vi "Wash Display Console View.vi"(8 "error in (no error)":errorcluster, 11 "View Model":T2) -> (0 "error out":errorcluster)   [LabVIEW 2017]
doc: "The interface via wich the wash controller displays the progres of the car wash.\n[Covers: UI3]"
uses:
  View Model/Controls/View Model.ctl
  View Model/Controls/Shared Model.ctl
  Error Handler/Controls/Error Model.ctl
  Error Handler/Controls/Error Data.ctl
  Error Handler/Controls/Error Level.ctl
  Configuration/Controls/Config Model.ctl
  Configuration/Controls/Config Record.ctl
  Configuration/Controls/Config Data.ctl
  Configuration/Controls/Config Command.ctl
  Controller/Controls/Controler Model.ctl
  Entry Console View/Controls/Entry Console - Wash Steps.ctl
  Controller/Controls/Controller - Overhead.ctl
  Controller/Controls/Controller - States.ctl
  Controller/Controls/Controller - Wash Step.ctl
  Vehicle Position View/Controls/Vehicle - Station Enum.ctl
  Controller/Controls/Controller - Event.ctl
  Controller/Controls/Controller - Commands.ctl
panel:
  out "Time Remaining":dbl format="%07.2g"
  out "Wash Entry":bool
  out "Vehicle Out of Position":bool
  out "Car Wash Indicators":T1
  # "Seconds"
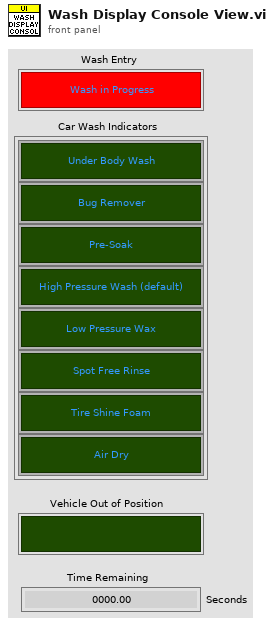
[diagram p1: front panel]
types:
  T1 = typedef "Entry Console - Wash Steps.ctl" = cluster{"Under Body Wash":bool, "Bug Remover":bool, "Pre-Soak":bool, "High Pressure Wash":bool, "Low Pressure Wax":bool, "Spot Free Rinse":bool, "Tire Shine Foam":bool, "Air Dry":bool}
  T2 = typedef "View Model.ctl" = cluster{"Shared Model":T3, "Error Model":T4, "Config Model":T5, "Controler Model":T6}
  T3 = typedef "Shared Model.ctl" = cluster{"Stop":refnum<user-event>, "Stop DVR":refnum<data-value>}
  T4 = typedef "Error Model.ctl" = cluster{"Error":refnum<user-event>}
  T5 = typedef "Config Model.ctl" = cluster{"Config Recs DVR":refnum<data-value>, "Config Data":refnum<user-event>, "Config Lock":refnum<user-event>, "Config Lock DVR":refnum<data-value>}
  T6 = typedef "Controler Model.ctl" = cluster{"Wash Step Exec":refnum<user-event>, "Wash Step Complete":refnum<user-event>, "Wash Cycle Complete":refnum<user-event>, "Wash Cycle Start":refnum<user-event>, "Vehicle Out of Position":refnum<user-event>, "Overhead DVR":refnum<data-value>, "Start Wash Step":refnum<user-event>, "Station Change":refnum<user-event>, "Command":refnum<user-event>}
  T7 = typedef "Controller - Wash Step.ctl" = enum16{"Under Body Wash", "Bug Remover", "Pre-Soak", "High Pressure Wash", "Low Pressure Wax", "Spot Free Rinse", "Tire Shine Foam", "Air Dry"}
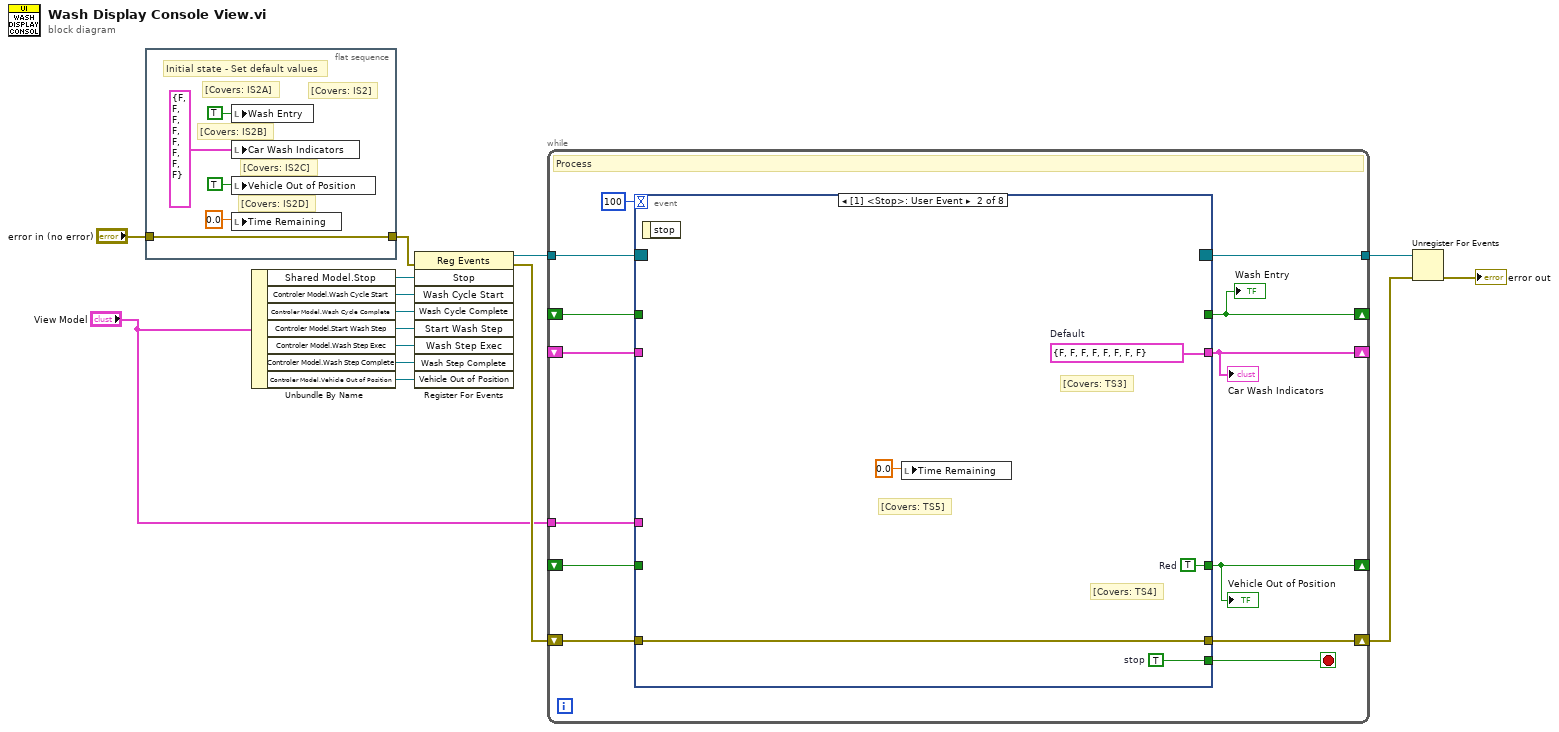
[diagram p0: block diagram]
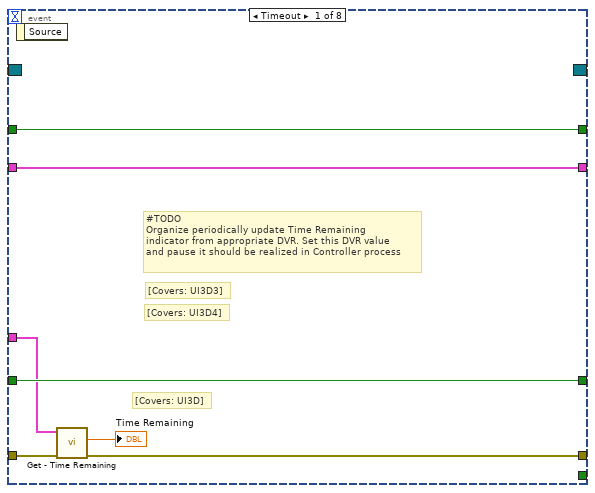
[diagram p2: hidden frame]
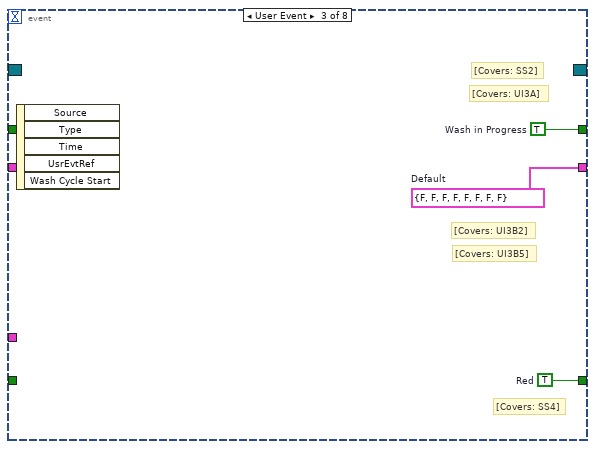
[diagram p3: hidden frame]
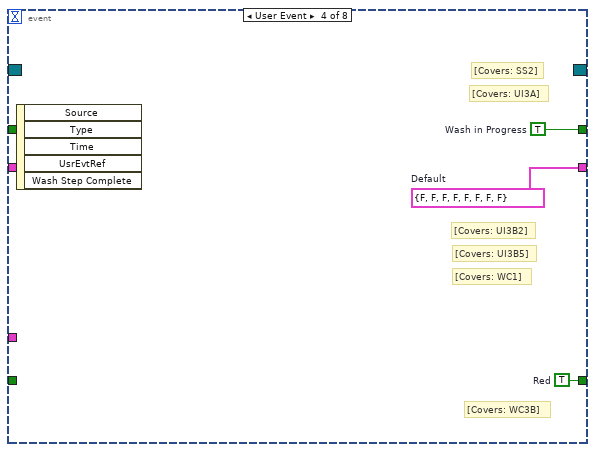
[diagram p4: hidden frame]
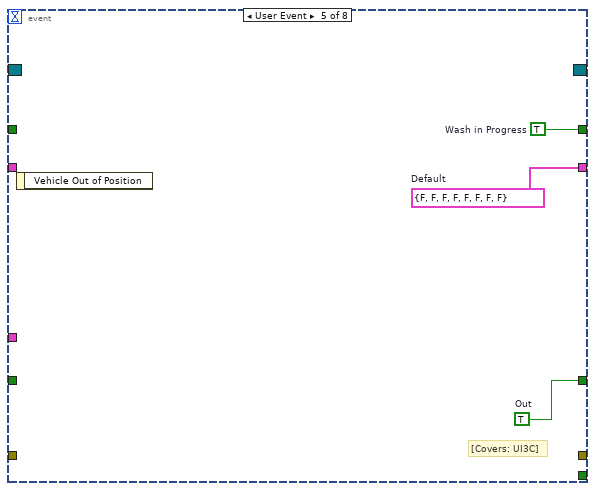
[diagram p5: hidden frame]
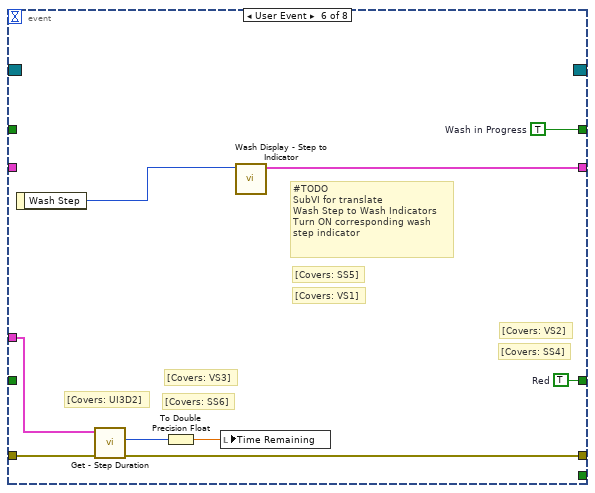
[diagram p6: hidden frame]
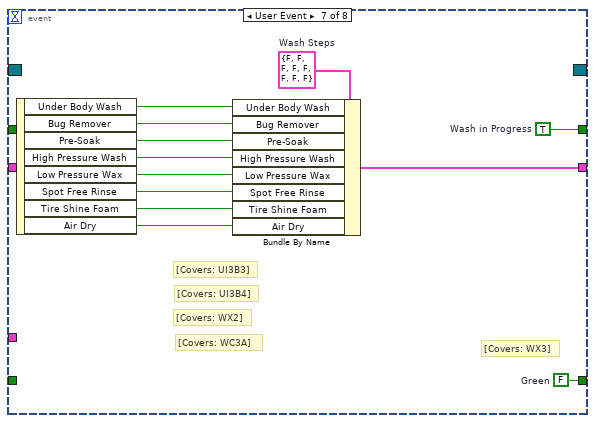
[diagram p7: hidden frame]
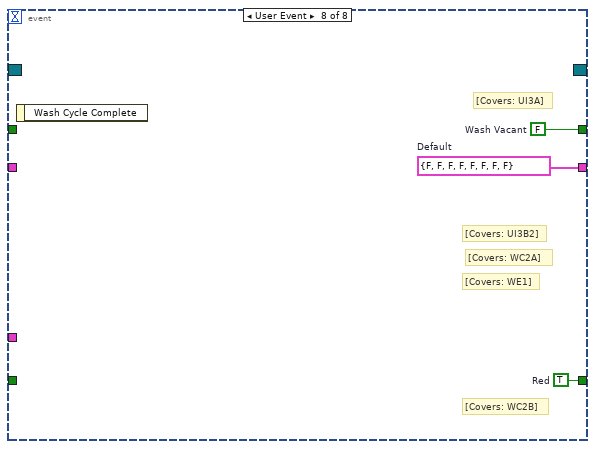
[diagram p8: hidden frame]
diagram:
  n1 = flat-sequence {
    tunnel: "error in (no error)" -> [w20]
    tunnel: [w20] -> w1
    frame #0 {
      # "[Covers: IS2D]"
      # "[Covers: IS2C]"
      # "[Covers: IS2B]"
      # "[Covers: IS2A]"
      # "[Covers: IS2]"
      # "Initial state - Set default values"
      n2 = local write "Wash Entry"(TRUE ("Wash Entry")) -> ()
      n3 = local write "Car Wash Indicators"(T1 {"Under Body Wash"=FALSE, "Bug Remover"=FALSE, "Pre-Soak"=FALSE, "High Pressure Wash"=FALSE, "Low Pressure Wax"=FALSE, "Spot Free Rinse"=FALSE, "Tire Shine Foam"=FALSE, "Air Dry"=FALSE} ("Car Wash Indicators")) -> ()
      n4 = local write "Vehicle Out of Position"(TRUE ("Vehicle Out of Position")) -> ()
      n5 = local write "Time Remaining"(0.0 ("Time Remaining")) -> ()
    }
  }
  n6 = Unbundle By Name("View Model") -> ("Shared Model.Stop"=w15:refnum<user-event>, "Controler Model.Wash Cycle Start"=w8:refnum<user-event>, "Controler Model.Wash Cycle Complete"=w7:refnum<user-event>, "Controler Model.Start Wash Step"=w4:refnum<user-event>, "Controler Model.Wash Step Exec"=w5:refnum<user-event>, "Controler Model.Wash Step Complete"=w6:refnum<user-event>, "Controler Model.Vehicle Out of Position"=w3:refnum<user-event>)
  n7 = register-events(error in=w1, w15, w8, w7, w4, w5, w6, w3) -> (reference out=w14:refnum<event-registration>, error out=w13:errorcluster)  [unwired: 1 in]
  n8 = while {
    tunnel: w14 -> [w33]
    shift-right: [w31] -> w11
    shift-left: w13 -> [w32]
    tunnel: [w29] -> w12
    tunnel: "View Model" -> [w28]
    shift-right: [w25] -> _
    shift-left: _ -> [w24]
    shift-right: [w26] -> _
    shift-left: _ -> [w23]
    shift-right: [w22] -> _
    shift-left: _ -> [w21]
    stop <- w30 stop-if-true
    # "Process"
    n9 = event shown="[1] <Stop>: User Event" {
      selector: w33 -> [_ _ _ _ _ _ _ _]
      dyn-events: [_ _ _ _ _ _ _ _] -> w29
      timeout: 100 -> [_ _ _ _ _ _ _ _]
      tunnel: w32 -> [w37 w45 _ _ _ w61 _ _]
      tunnel: [w36 w45 _ _ _ w58 _ _] -> w31
      tunnel: [_ w44 _ _ _ _ _ _] -> w30
      tunnel: w28 -> [w35 _ _ _ _ w60 _ _]
      tunnel: [w39 _ w48 w51 w54 w63 w75 w78] -> w26
      tunnel: [w40 w43 w47 w50 w53 w56 w65 w77] -> w25
      tunnel: [w38 w42 w46 w49 w52 w55 w64 w76] -> w22
      tunnel: w24 -> [w40 _ _ _ _ _ _ _]
      tunnel: w23 -> [w39 _ _ _ _ _ _ _]
      tunnel: w21 -> [w38 _ _ _ _ _ _ _]
      event Timeout {
        # "[Covers: UI3D]"
        # "[Covers: UI3D4]"
        # "[Covers: UI3D3]"
        # "#TODO\nOrganize periodically update Time Remaining\nindicator from appropriate DVR. Set this DVR value\nand pause it should be realized in Controller process"
        n10 = event-data() -> ()  [unwired: 1 in, 1 out]
        n11 = call "Get - Time Remaining.vi"("error in (no error)"=w37, "View Model"=w35) -> ("error out"=w36:errorcluster, "Elapsed Time"=→"Time Remaining":dbl)  [unwired: 7 in, 1 out]
      }
      event User Event {
        w42 = TRUE  # Red
        w43 = T1 {"Under Body Wash"=FALSE, "Bug Remover"=FALSE, "Pre-Soak"=FALSE, "High Pressure Wash"=FALSE, "Low Pressure Wax"=FALSE, "Spot Free Rinse"=FALSE, "Tire Shine Foam"=FALSE, "Air Dry"=FALSE}  # Default
        w44 = TRUE  # stop
        # "[Covers: TS5]"
        # "[Covers: TS4]"
        # "[Covers: TS3]"
        n12 = event-data() -> ()  [unwired: 1 in, 1 out]
        n13 = local write "Time Remaining"(0.0 ("Time Remaining")) -> ()
      }
      event User Event {
        w46 = TRUE  # Red
        w47 = T1 {"Under Body Wash"=FALSE, "Bug Remover"=FALSE, "Pre-Soak"=FALSE, "High Pressure Wash"=FALSE, "Low Pressure Wax"=FALSE, "Spot Free Rinse"=FALSE, "Tire Shine Foam"=FALSE, "Air Dry"=FALSE}  # Default
        w48 = TRUE  # Wash in Progress
        # "[Covers: SS4]"
        # "[Covers: SS2]"
        # "[Covers: UI3B5]"
        # "[Covers: UI3B2]"
        # "[Covers: UI3A]"
        n14 = event-data() -> ()  [unwired: 1 in, 5 out]
      }
      event User Event {
        w49 = TRUE  # Red
        w50 = T1 {"Under Body Wash"=FALSE, "Bug Remover"=FALSE, "Pre-Soak"=FALSE, "High Pressure Wash"=FALSE, "Low Pressure Wax"=FALSE, "Spot Free Rinse"=FALSE, "Tire Shine Foam"=FALSE, "Air Dry"=FALSE}  # Default
        w51 = TRUE  # Wash in Progress
        # "[Covers: WC3B]"
        # "[Covers: WC1]"
        # "[Covers: SS2]"
        # "[Covers: UI3B5]"
        # "[Covers: UI3B2]"
        # "[Covers: UI3A]"
        n15 = event-data() -> ()  [unwired: 1 in, 5 out]
      }
      event User Event {
        w52 = TRUE  # Out
        w53 = T1 {"Under Body Wash"=FALSE, "Bug Remover"=FALSE, "Pre-Soak"=FALSE, "High Pressure Wash"=FALSE, "Low Pressure Wax"=FALSE, "Spot Free Rinse"=FALSE, "Tire Shine Foam"=FALSE, "Air Dry"=FALSE}  # Default
        w54 = TRUE  # Wash in Progress
        # "[Covers: UI3C]"
        n16 = event-data() -> ()  [unwired: 1 in, 1 out]
      }
      event User Event {
        w55 = TRUE  # Red
        w63 = TRUE  # Wash in Progress
        # "[Covers: VS3]"
        # "[Covers: VS2]"
        # "[Covers: VS1]"
        # "[Covers: SS4]"
        # "[Covers: SS5]"
        # "#TODO\nSubVI for translate\nWash Step to Wash Indicators\nTurn ON corresponding wash \nstep indicator"
        # "[Covers: SS6]"
        # "[Covers: UI3D2]"
        n17 = event-data() -> ("Wash Step"=w57:T7)  [unwired: 1 in]
        n18 = call "Get - Step Duration.vi"("error in (no error)"=w61, "View Model"=w60) -> ("error out"=w58:errorcluster, "Step Duration"=w59:u32)  [unwired: 7 in, 1 out]
        n19 = To Double Precision Float(number=w59) -> (double precision float=w62:dbl)
        n20 = local write "Time Remaining"(w62) -> ()
        n21 = call "Wash Display - Step to Indicator.vi"("Wash Step"=w57) -> ("Wash Steps"=w56:T1)  [unwired: 9 in, 1 out]
      }
      event User Event {
        w64 = FALSE  # Green
        w74 = T1 {"Under Body Wash"=FALSE, "Bug Remover"=FALSE, "Pre-Soak"=FALSE, "High Pressure Wash"=FALSE, "Low Pressure Wax"=FALSE, "Spot Free Rinse"=FALSE, "Tire Shine Foam"=FALSE, "Air Dry"=FALSE}  # Wash Steps
        w75 = TRUE  # Wash in Progress
        # "[Covers: WC3A]"
        # "[Covers: WX3]"
        # "[Covers: WX2]"
        # "[Covers: UI3B4]"
        # "[Covers: UI3B3]"
        n22 = event-data() -> ("Under Body Wash"=w73:bool, "Bug Remover"=w66:bool, "Pre-Soak"=w67:bool, "High Pressure Wash"=w68:bool, "Low Pressure Wax"=w69:bool, "Spot Free Rinse"=w70:bool, "Tire Shine Foam"=w71:bool, "Air Dry"=w72:bool)  [unwired: 1 in]
        n23 = Bundle By Name(cluster=w74, "Under Body Wash"=w73, "Bug Remover"=w66, "Pre-Soak"=w67, "High Pressure Wash"=w68, "Low Pressure Wax"=w69, "Spot Free Rinse"=w70, "Tire Shine Foam"=w71, "Air Dry"=w72) -> (w65:T1)
      }
      event User Event {
        w76 = TRUE  # Red
        w77 = T1 {"Under Body Wash"=FALSE, "Bug Remover"=FALSE, "Pre-Soak"=FALSE, "High Pressure Wash"=FALSE, "Low Pressure Wax"=FALSE, "Spot Free Rinse"=FALSE, "Tire Shine Foam"=FALSE, "Air Dry"=FALSE}  # Default
        w78 = FALSE  # Wash Vacant
        # "[Covers: WE1]"
        # "[Covers: WC2B]"
        # "[Covers: WC2A]"
        # "[Covers: UI3B2]"
        # "[Covers: UI3A]"
        n24 = event-data() -> ()  [unwired: 1 in, 1 out]
      }
    }
    "Wash Entry" <- w26
    "Car Wash Indicators" <- w25
    "Vehicle Out of Position" <- w22
  }
  n25 = Unregister For Events(event registration refnum=w12, error in=w11) -> (error out=→"error out":errorcluster)
